vi "CalcSubbandgapTemp.vi"(0 "Voltage 2":dbl, 1 "Voltage 1":dbl) -> (3 "Voltage 1":dbl, 4 "Voltage2":dbl, 5 "Kelvin":dbl format="%#.6g", 6 "Celcius":dbl format="%#.6g")   [LabVIEW 2009]
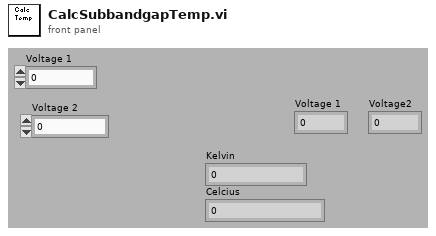
[diagram p1: front panel]
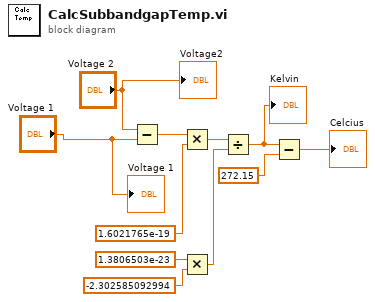
[diagram p0: block diagram]
diagram:
  n1 = Subtract(x="Voltage 2", y="Voltage 1") -> (x-y=w3:dbl)
  n2 = Multiply(x=w3, y=1.6021765e-19) -> (x*y=w7:dbl)
  n3 = Multiply(x=1.3806503e-23, y=-2.302585092994) -> (x*y=w8:dbl)
  n4 = Divide(x=w7, y=w8) -> (x/y=w9:dbl)
  "Kelvin" <- w9
  n5 = Subtract(x=w9, y=272.15) -> (x-y=→"Celcius":dbl)
  "Voltage2" <- "Voltage 2"
  "Voltage 1" <- "Voltage 1"
